vi "accesstoken.vi"(8 "error in (no error)":errorcluster caption="错误输入（无错误）", 11 "HTTP发送 输入":refnum<class "HTTP发送.lvclass">) -> (0 "error out":errorcluster caption="错误输出", 3 "HTTP发送 输出":refnum<class "HTTP发送.lvclass">)   [LabVIEW 2022 SP3, in "工况数据上传.lvlib" / "HTTP发送.lvclass"]
uses:
  <vilib>/httpClient/POSTBuffer.vi
  <vilib>/httpClient/LabVIEWHTTPClient.lvlib
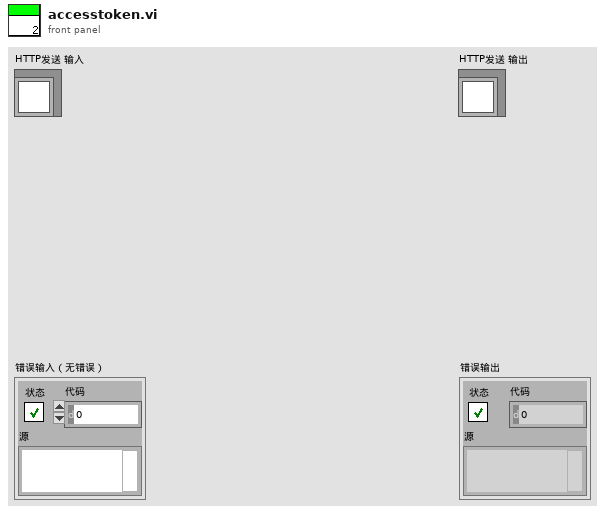
[diagram p1: front panel]
types:
  T1 = cluster{"code":string, "message":string, "timestamp":u64, "success":bool}
  T2 = cluster{"url":string, "loginTokenRequest":cluster{"clientId":string, "clientSecret":string, "grantType":string, "password":string, "scope":string, "userName":string, "userType":string}, "自动获取MN":bool}
  T3 = cluster{"clientId":string, "clientSecret":string, "grantType":string, "password":string, "scope":string, "userName":string, "userType":string}
  T4 = typedef "LabVIEWHTTPClient.lvlib/ClientHandle.ctl" = refnum<k1>
  T5 = cluster{"code":string, "message":string, "timestamp":u64, "data":cluster{"bearerType":string, "oauth2Type":string, "accessToken":string, "tokenType":string, "expiresIn":u64, "refreshToken":string, "scope":string[], "tokenDetail":cluster{"dataSource":string, "username":string, "userId":string, "userType":string, "enabled":bool, "accountNonExpired":bool, "credentialsNonExpired":bool, "accountNonLocked":bool}}, "success":bool}
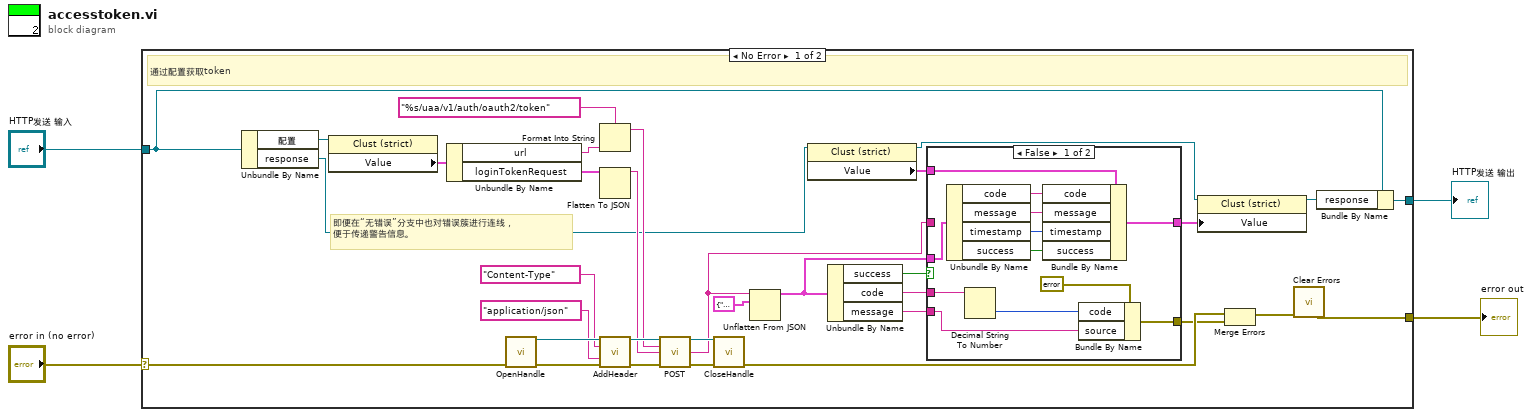
[diagram p0: block diagram]
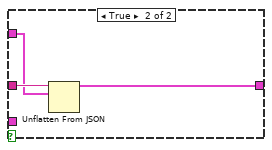
[diagram p2: hidden frame]
diagram:
  n1 = case shown="No Error" "error in (no error)" {
    selector: "error in (no error)" -> [w16 w54]
    tunnel: [w5 w54] -> w3
    tunnel: [w8 w53] -> w1
    tunnel: "HTTP发送 输入" -> [w9 w53]
    frame No Error {
      # "即便在“无错误”分支中也对错误簇进行连线，\n便于传递警告信息。"
      # "通过配置获取token"
      n2 = Unbundle By Name(w9) -> ("配置"=w13:refnum<vi>, "response"=w15:refnum<vi>)
      n3 = property class="Clust (strict)"(reference=w13) -> ("Value"=w12:T2)  [unwired: 1 in, 2 out]
      n4 = Unbundle By Name(w12) -> ("url"=w25:string, "loginTokenRequest"=w28:T3)
      n5 = call <vilib>:"OpenHandle.vi"("error in (no error)"=w16) -> ("client handle out"=w37:T4, "error out"=w35:errorcluster)  [unwired: 13 in]
      n6 = Format Into String(format string="%s/uaa/v1/auth/oauth2/token" ("url"), w25) -> (resulting string=w27:string)  [unwired: 2 in, 1 out]
      n7 = Flatten To JSON(anything=w28) -> (JSON string=w29:string)  [unwired: 2 in, 1 out]
      n8 = call <vilib>:"AddHeader.vi"("client handle"=w37, "header"="Content-Type", "value"="application/json", "error in (no error)"=w35) -> ("client handle out"=w33:T4, "error out"=w32:errorcluster)  [unwired: 10 in]
      n9 = call-poly <vilib>:"POST.vi"("client handle"=w33, "url"=w27, "buffer"=w29, "error in (no error)"=w32) -> ("client handle out"=w31:T4, "body"=w22:string, "error out"=w30:errorcluster)  [unwired: 8 in, 1 out]
      n10 = call <vilib>:"CloseHandle.vi"("client handle"=w31, "error in (no error)"=w30) -> ("error out"=w19:errorcluster)  [unwired: 13 in]
      n11 = Unflatten From JSON(JSON string=w22, type and defaults=T1 {"code"="", "message"="", "timestamp"=0, "success"=FALSE} ("response 2")) -> (value=w21:T1)  [unwired: 5 in, 1 out]
      n12 = property class="Clust (strict)"(reference=w15) -> (reference out=w11:refnum<vi>, "Value"=w14:T5)  [unwired: 1 in, 1 out]
      n13 = Unbundle By Name(w21) -> ("success"=w23:bool, "code"=w17:string, "message"=w20:string)
      n14 = case shown="False" w23 {
        tunnel: [w49 w52] -> w10
        tunnel: w22 -> [_ w51]
        tunnel: w21 -> [w48 _]
        tunnel: w20 -> [w42 _]
        tunnel: [w41 _] -> w18
        tunnel: w17 -> [w40 _]
        tunnel: w14 -> [w38 w50]
        frame False {
          n15 = Unbundle By Name(w48) -> ("code"=w47:string, "message"=w46:string, "timestamp"=w45:u64, "success"=w44:bool)
          n16 = Decimal String To Number(string=w40) -> (number=w39:i32)  [unwired: 2 in, 1 out]
          n17 = Bundle By Name(cluster=w38, "code"=w47, "message"=w46, "timestamp"=w45, "success"=w44) -> (w49:T5)
          n18 = Bundle By Name(cluster=errorcluster {"status"=TRUE, "code"=0, "source"=""} ("错误常量"), "code"=w39, "source"=w42) -> (w41:errorcluster)
        }
        frame True {
          n19 = Unflatten From JSON(JSON string=w51, type and defaults=w50) -> (value=w52:T5)  [unwired: 5 in, 1 out]
        }
      }
      n20 = property class="Clust (strict)"(reference=w11, "Value"=w10) -> (reference out=w7:refnum<vi>)  [unwired: 1 in, 1 out]
      n21 = Merge Errors(w19, w18) -> (w6:errorcluster)
      n22 = call <vilib>:"Clear Errors.vi"("error in (no error)"=w6) -> ("error out"=w5:errorcluster)  [unwired: 5 in, 1 out]
      n23 = Bundle By Name(cluster=w9, "response"=w7) -> (w8:refnum<class "HTTP发送.lvclass">)
    }
    frame Error {
    }
  }
  "error out" <- w3
  "HTTP发送 输出" <- w1
